vi "Read Message Status.vi"(8 "error in (no error)":errorcluster, 11 "CS++Message in":refnum<class "CS++Message.lvclass">) -> (0 "error out":errorcluster, 2 "Message Status":T1 items=["Simple", "Dialog", "PVUpdate", "Dialog + PVUpdate", "N/A", "Unknown"], 3 "CS++Message out":refnum<class "CS++Message.lvclass">)   [LabVIEW 2015, in "CS++Message.lvlib" / "CS++Message.lvclass"]
uses:
  CS++Message.lvclass
  MessageStatus.ctl
  CS++Message.lvclass/CS++Message.ctl
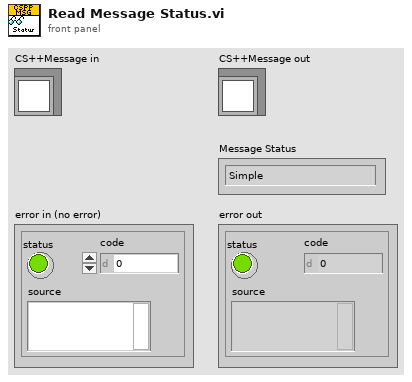
[diagram p1: front panel]
types:
  T1 = typedef "CS++Message.lvlib/CS++Message.lvclass/MessageStatus.ctl" = u16
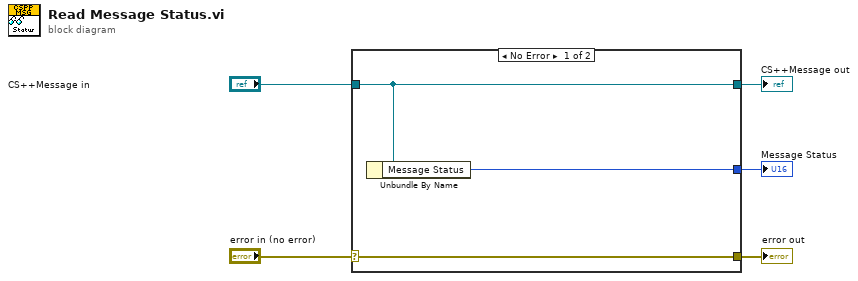
[diagram p0: block diagram]
diagram:
  n1 = case shown="No Error" "error in (no error)" {
    selector: "error in (no error)" -> [w8 w9]
    tunnel: [w8 w9] -> w4
    tunnel: [w7 w10] -> w2
    tunnel: "CS++Message in" -> [w7 w10]
    tunnel: [w6 _] -> w1
    frame No Error {
      n2 = Unbundle By Name(w7) -> ("Message Status"=w6:T1)
    }
    frame Error {
    }
  }
  "error out" <- w4
  "CS++Message out" <- w2
  "Message Status" <- w1
